vi "Finish Calibration.vi"(8 "Error in":errorcluster caption="Error in (no error)", 9 "Position":u32, 10 "Cree Comms in":refnum<class "Cree Communications.lvclass">, 11 "Calibration in":refnum<class "Calibration.lvclass">) -> (0 "error out":errorcluster)   [LabVIEW 2015, in "Calibration.lvclass"]
uses:
  Calibration.lvclass
  Classes/Cree Communications/Class/Cree Communications.lvclass
  Classes/Cree Communications/Cree Comms Messages/Set Lock Byte/Set Lock Byte.lvclass
  Classes/Cree Communications/Cree Comms Messages/Write Calibration Mode/Set Calibration Mode.lvclass
  Classes/Cree Communications/Cree Comms Messages/Set Test Mode/Set Test Mode.lvclass
  Classes/Cree Communications/Cree Comms Messages/CC Message/CC Message.lvclass/CC Message.ctl
  Classes/Cree Communications/Cree Comms Messages/CC Message/CC Message.lvclass
  <vilib>/Cree, Inc/Cree Test Framework/Classes/Base Objects/Base Class/Base Class/Base Class.lvclass
  Driver Test/Driver Test.lvclass
  Classes/Application/Class/Application.lvclass
  Test Class/Test Class.lvclass
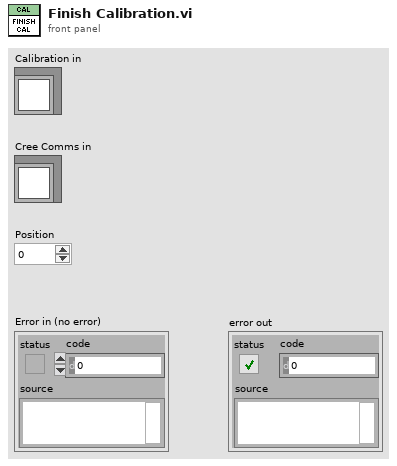
[diagram p1: front panel]
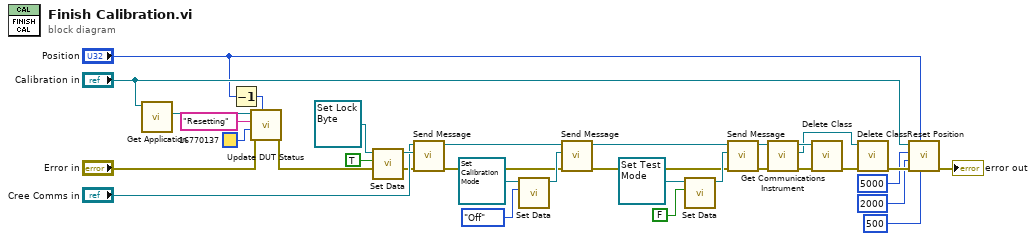
[diagram p0: block diagram]
diagram:
  n1 = call "Get Application.vi"("Test Class in"="Calibration in") -> ("Application.lvlib:Application.lvclass"=w15:refnum<class "Application.lvclass">)  [unwired: 9 in, 1 out]
  n2 = Decrement(x="Position") -> (x-1=w10:u32)
  n3 = call "Update DUT Status.vi"("Position"=w10, "error in (no error)"="Error in", "BG Color"=u32 16770137, "Message ('')"="Resetting", "Application in"=w15) -> ("error out"=w8:errorcluster)  [unwired: 5 in, 1 out]
  n4 = call "Set Data.vi"("Data"=TRUE ("Message Type"), "CC Message in"=refnum<class "Set Lock Byte.lvclass"> refnum ("Cree Comms Messages.lvlib:Set Lock Byte.lvclass")) -> ("CC Message out"=w33:refnum<class "Set Lock Byte.lvclass">)  [unwired: 8 in, 1 out]
  n5 = call "Send Message.vi"("error in (no error)"=w8, "Cree Comms Message"=w33, "Acrobat Template in"="Cree Comms in") -> ("error out"=w18:errorcluster, "Acrobat Template out"=w19:refnum<class "Cree Communications.lvclass">)  [unwired: 7 in]
  n6 = call "Set Data.vi"("Data"=enum8{"Off", "On", "<Invalid>"}."Off" ("Message Type"), "CC Message in"=refnum<class "Set Calibration Mode.lvclass"> refnum ("Cree Comms Messages.lvlib:Set Calibration Mode.lvclass")) -> ("CC Message out"=w20:refnum<class "Set Calibration Mode.lvclass">)  [unwired: 8 in, 1 out]
  n7 = call "Send Message.vi"("error in (no error)"=w18, "Cree Comms Message"=w20, "Acrobat Template in"=w19) -> ("error out"=w3:errorcluster, "Acrobat Template out"=w4:refnum<class "Cree Communications.lvclass">)  [unwired: 7 in]
  n8 = call "Set Data.vi"("Data"=FALSE ("Message Type"), "CC Message in"=refnum<class "Set Test Mode.lvclass"> refnum ("Cree Comms Messages.lvlib:Set Test Mode.lvclass")) -> ("CC Message out"=w5:refnum<class "Set Test Mode.lvclass">)  [unwired: 8 in, 1 out]
  n9 = call "Send Message.vi"("error in (no error)"=w3, "Cree Comms Message"=w5, "Acrobat Template in"=w4) -> ("error out"=w2:errorcluster, "Acrobat Template out"=w1:refnum<class "Cree Communications.lvclass">)  [unwired: 7 in]
  n10 = call "Get Communications Instrument.vi"("error in (no error)"=w2, "Cree Communications in"=w1) -> ("error out"=w27:errorcluster, "Communication Instrument"=w26:refnum<class "Comm Instrument.lvclass">, "Cree Communications out"=w29:refnum<class "Cree Communications.lvclass">)  [unwired: 7 in]
  n11 = call <vilib>:"Delete Class.vi"("error in (no error)"=w27, "Base Class in"=w29) -> ("error out"=w28:errorcluster)  [unwired: 8 in, 1 out]
  n12 = call <vilib>:"Delete Class.vi"("error in (no error)"=w28, "Base Class in"=w26) -> ("error out"=w25:errorcluster)  [unwired: 8 in, 1 out]
  n13 = call "Reset Position.vi"("Wait Before Reset (0ms)"=u32 500 ("Wait After Power Off (1500 ms)"), "Position"="Position", "error in (no error)"=w25, "Wait After Power On (500 ms)"=u32 2000 ("Wait After Power Off (1500 ms)"), "Wait After Power Off (1500 ms)"=u32 5000, "Driver Test"="Calibration in") -> ("error out"=→"error out":errorcluster)  [unwired: 5 in]
